vi "UpdateRepo.vi"(11 "package":path) -> (3 "package out":path)   [LabVIEW 2014, in "Raspberry Pi Compatible Compiler for LabVIEW.lvlib" / "Python Functions.lvlib"]
uses:
  Python Functions.lvlib
panel:
  out "standard output":string
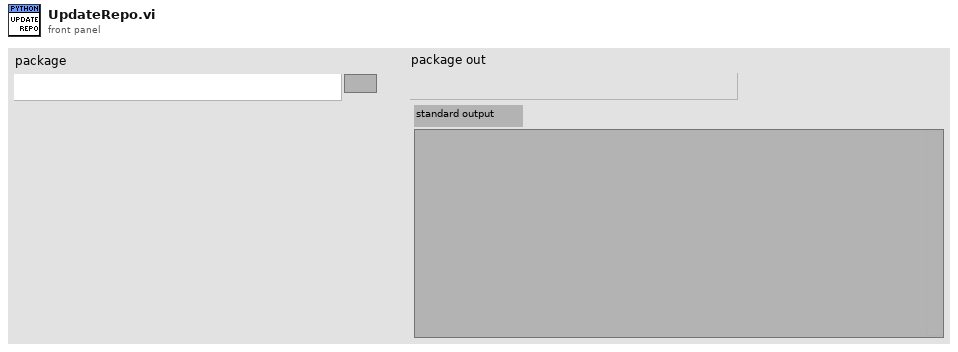
[diagram p1: front panel]
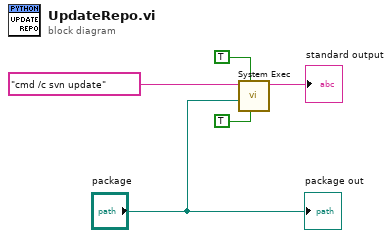
[diagram p0: block diagram]
diagram:
  n1 = call <vilib>:"System Exec.vi"("run minimized? (F)"=TRUE, "wait until completion? (T)"=TRUE, "working directory"="package", "command line"="cmd /c svn update" ("standard input")) -> ("standard output"=→"standard output":string)  [unwired: 4 in, 3 out]
  "package out" <- "package"
